vi "OBJ_MAIN_get_test_data.vi"(8 "error_in":errorcluster, 11 "all_config_info":T1 {"main_ini_file"."MD-R Flow control" items=["None"=0, "XON/XOFF"=1, "RTS/CTS"=2, "DTR/DSR"=4]; "main_ini_file"."MD-R Stop bits" items=["1.0"=10, "1.5"=15, "2.0"=20]; "main_ini_file"."MD-L Flow control" items=["None"=0, "XON/XOFF"=1, "RTS/CTS"=2, "DTR/DSR"=4]; "main_ini_file"."MD-L Stop bits" items=["1.0"=10, "1.5"=15, "2.0"=20]; "main_ini_file"."SCANNER Flow control" items=["None"=0, "XON/XOFF"=1, "RTS/CTS"=2, "DTR/DSR"=4]; "main_ini_file"."SCANNER Stop bits" items=["1.0"=10, "1.5"=15, "2.0"=20]}) -> (0 "error_out":errorcluster, 1 "Timed out?":bool, 2 "measurement_right":string, 3 "measurement_left":string)   [LabVIEW 2020]
uses:
  ini/typedef/OBJ_all_config_info.ctl
  ini/typedef/OBJ_main_ini_file.ctl
  queues/typedef/OBJ_queue_refnums.ctl
  queues/typedef/OBJ_MAIN_queue_element.ctl
  OBJ_MAIN_sequence_state.ctl
  queues/typedef/OBJ_SCANNER_queue_element.ctl
  SCANNER/OBJ_SCANNER_sequence_state.ctl
  queues/typedef/OBJ_MD_queue_element.ctl
  MEASURING_DEVICE/OBJ_MD_sequence_state.ctl
  queues/typedef/OBJ_GUI_TIMER_queue_element.ctl
  GUI_TIMER/OBJ_GUI_TIMER_sequence_state.ctl
  FGV/error_buffer/FGV_OBJ_error_buffer.ctl
  OBJ_thread.ctl
  <vilib>/regexp/Match Regular Expression.xnode
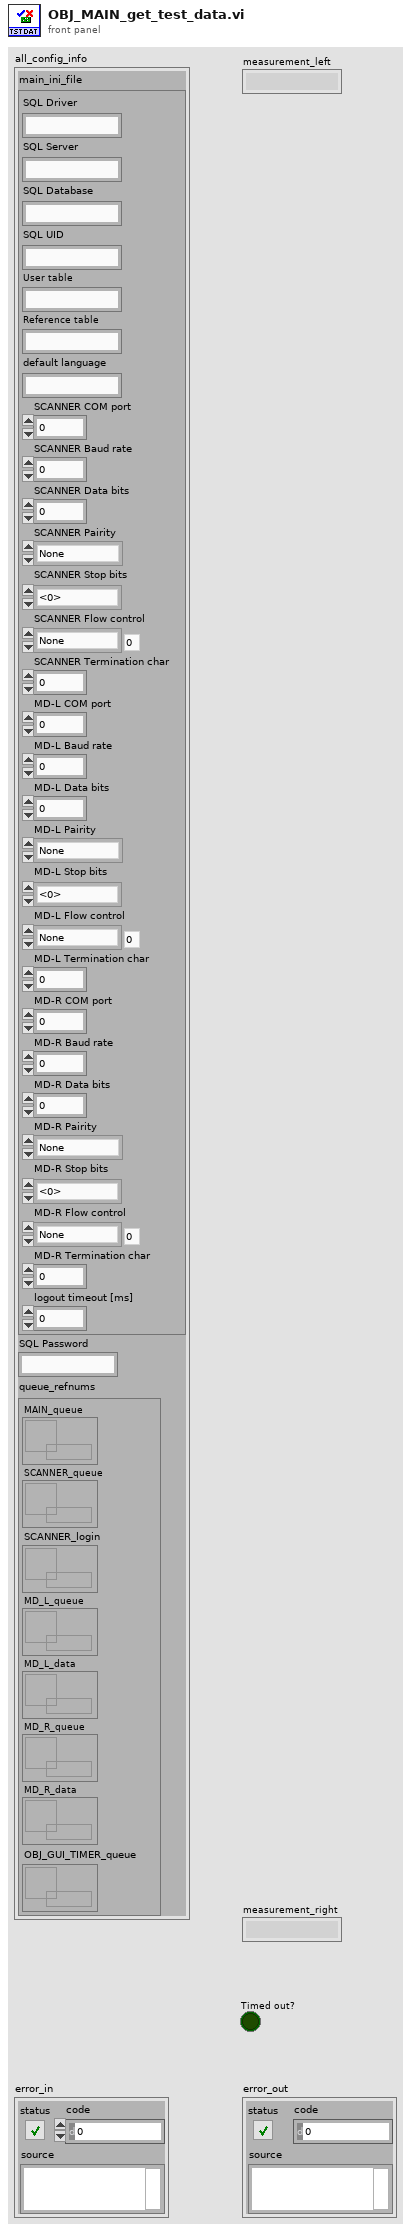
[diagram p1: front panel]
types:
  T1 = typedef "OBJ_all_config_info.ctl" = cluster{"main_ini_file":T2, "SQL Password":string, "queue_refnums":T3}
  T2 = typedef "OBJ_main_ini_file.ctl" = cluster{"SQL Driver":string, "SQL Server":string, "SQL Database":string, "SQL UID":string, "User table":string, "Reference table":string, "default language":string, "SCANNER COM port":u16, "SCANNER Baud rate":u32, "SCANNER Data bits":u16, "SCANNER Pairity":enum16{"None", "Odd", "Even", "Mark", "Space"}, "SCANNER Stop bits":u16, "SCANNER Flow control":u16, "SCANNER Termination char":u8, "MD-L COM port":u16, "MD-L Baud rate":u32, "MD-L Data bits":u16, "MD-L Pairity":enum16{"None", "Odd", "Even", "Mark", "Space"}, "MD-L Stop bits":u16, "MD-L Flow control":u16, "MD-L Termination char":u8, "MD-R COM port":u16, "MD-R Baud rate":u32, "MD-R Data bits":u16, "MD-R Pairity":enum16{"None", "Odd", "Even", "Mark", "Space"}, "MD-R Stop bits":u16, "MD-R Flow control":u16, "MD-R Termination char":u8, "logout timeout [ms]":i32}
  T3 = typedef "OBJ_queue_refnums.ctl" = cluster{"MAIN_queue":refnum<queue>, "SCANNER_queue":refnum<queue>, "SCANNER_login":refnum<queue>, "MD_L_queue":refnum<queue>, "MD_L_data":refnum<queue>, "MD_R_queue":refnum<queue>, "MD_R_data":refnum<queue>, "OBJ_GUI_TIMER_queue":refnum<queue>}
  T4 = typedef "OBJ_MD_queue_element.ctl" = cluster{"state":T5, "variable":variant}
  T5 = typedef "OBJ_MD_sequence_state.ctl" = enum16{"initialize", "get_next_state", "get_measurement", "error", "stop"}
  T6 = typedef "OBJ_thread.ctl" = enum16{"MAIN", "SCANNER", "MD - LEFT", "MD - RIGHT", "GUI TIMER"}
  T7 = typedef "FGV_OBJ_error_buffer.ctl" = enum16{"initialize", "clear", "display", "get_status"}
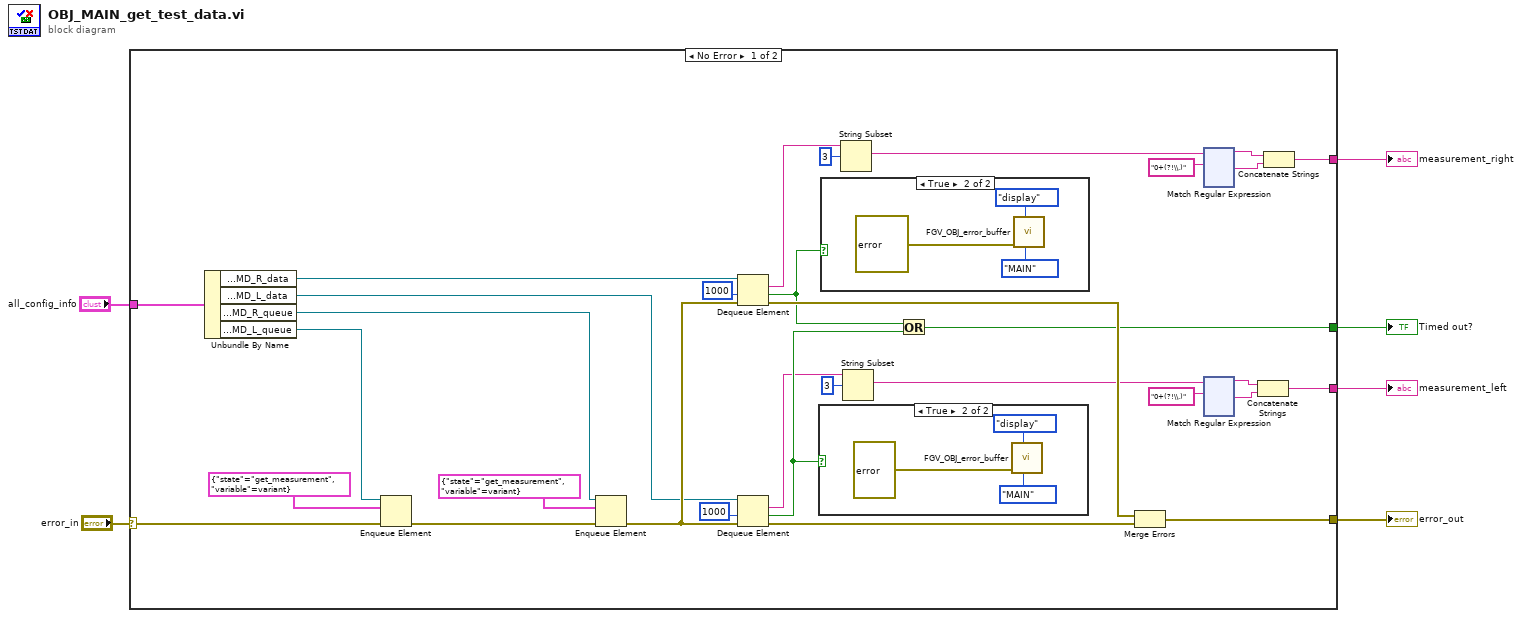
[diagram p0: block diagram]
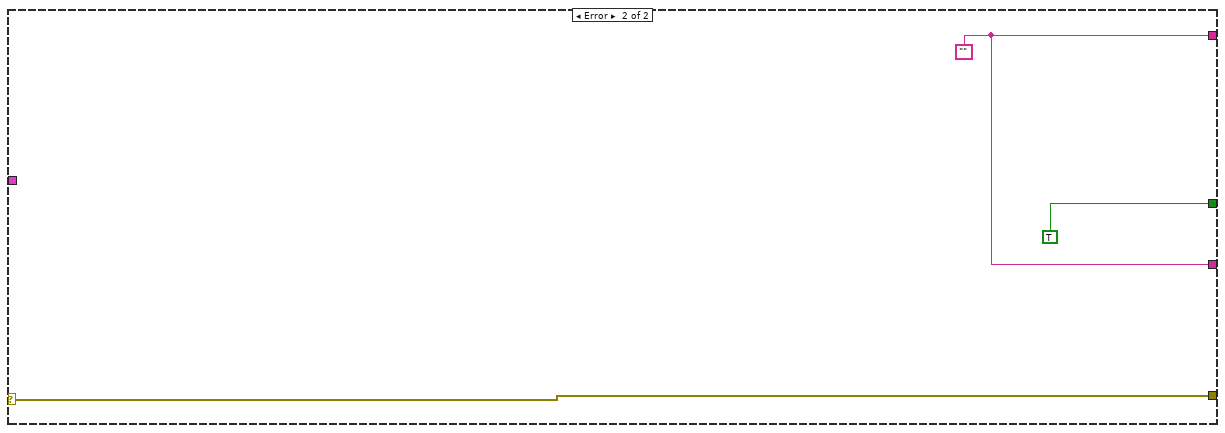
[diagram p4: hidden frame]
diagram:
  n1 = case shown="No Error" "error_in" {
    selector: "error_in" -> [w32 w275]
    tunnel: "all_config_info" -> [w33 _]
    tunnel: [w24 w275] -> w4
    tunnel: [w12 w273] -> w2
    tunnel: [w9 w273] -> w1
    tunnel: [w21 TRUE] -> w3
    frame No Error {
      n2 = Unbundle By Name(w33) -> ("queue_refnums.MD_R_data"=w27:refnum<queue>, "queue_refnums.MD_L_data"=w28:refnum<queue>, "queue_refnums.MD_R_queue"=w37:refnum<queue>, "queue_refnums.MD_L_queue"=w34:refnum<queue>)
      n3 = Enqueue Element(queue=w34, element=T4 {"state"=enum."get_measurement", "variable"=variant}, error in (no error)=w32) -> (error out=w36:errorcluster)  [unwired: 1 in, 2 out]
      n4 = Enqueue Element(queue=w37, element=T4 {"state"=enum."get_measurement", "variable"=variant}, error in (no error)=w36) -> (error out=w30:errorcluster)  [unwired: 1 in, 2 out]
      n5 = Dequeue Element(queue=w27, timeout in ms (-1)=1000, error in (no error)=w30) -> (element=w20:string, timed out?=w22:bool, error out=w26:errorcluster)  [unwired: 1 out]
      n6 = Dequeue Element(queue=w28, timeout in ms (-1)=1000, error in (no error)=w30) -> (element=w17:string, timed out?=w23:bool, error out=w25:errorcluster)  [unwired: 1 out]
      n7 = case shown="True" w23 {
        frame False {
        }
        frame True {
          n8 = call "FGV_OBJ_error_buffer.vi"("thread"=OBJ_thread."MAIN", "option"=FGV_OBJ_error_buffer."display", "error_in"=errorcluster {"status"=TRUE, "code"=91381, "source"="Timeout while waiting for data - measuring device - LEFT"}) -> ()  [unwired: 7 in, 2 out]
        }
      }
      n9 = case shown="True" w22 {
        frame False {
        }
        frame True {
          n10 = call "FGV_OBJ_error_buffer.vi"("thread"=OBJ_thread."MAIN", "option"=FGV_OBJ_error_buffer."display", "error_in"=errorcluster {"status"=TRUE, "code"=91380, "source"="Timeout while waiting for data - measuring device - RIGHT"}) -> ()  [unwired: 7 in, 2 out]
        }
      }
      n11 = String Subset(string=w20, offset (0)=3) -> (substring=w8:string)  [unwired: 1 in]
      n12 = String Subset(string=w17, offset (0)=3) -> (substring=w7:string)  [unwired: 1 in]
      n13 = Or(x=w22, y=w23) -> (x .or. y?=w21:bool)
      n14 = Merge Errors(w26, w25) -> (w24:errorcluster)
      n15 = xnode "Match Regular Expression"("input string"=w8, "regular expression"="0+(?!\\.)") -> ("before match"=w14:string, "after match"=w13:string)  [unwired: 4 in, 3 out]
      n16 = xnode "Match Regular Expression"("input string"=w7, "regular expression"="0+(?!\\.)") -> ("before match"=w11:string, "after match"=w10:string)  [unwired: 4 in, 3 out]
      n17 = Concatenate Strings(w11, w10) -> (w9:string)
      n18 = Concatenate Strings(w14, w13) -> (w12:string)
    }
    frame Error {
      w273 = ""
    }
  }
  "error_out" <- w4
  "Timed out?" <- w3
  "measurement_right" <- w2
  "measurement_left" <- w1
